vi "U8_3_byte_Array_with_dividor.vi"(10 "Array In":u8[](array[numeric]), 11 "Nmbr_of_datasamples":dbl=128.0) -> (0 "Current":dbl[](graph), 1 "mV":dbl, 2 "Voltage":dbl[](graph), 3 "Loop count":dbl, 4 "COM":dbl[](graph), 6 "HEXVAL":string)   [LabVIEW 2012]
panel:
  out "Dividor Value":dbl[](array[numeric])
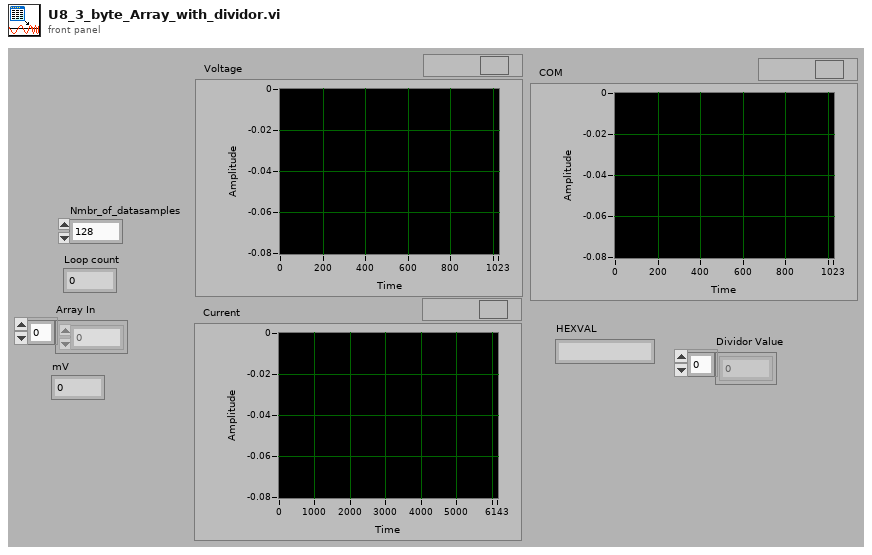
[diagram p1: front panel]
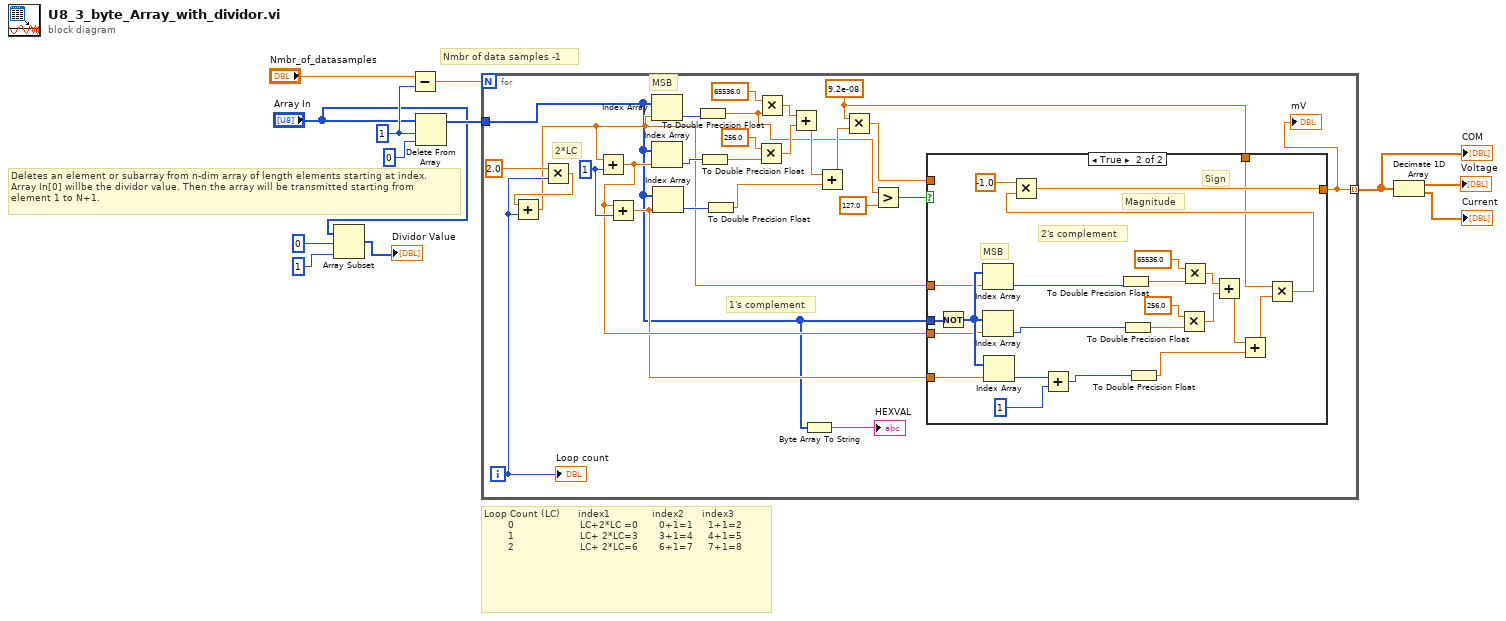
[diagram p0: block diagram]
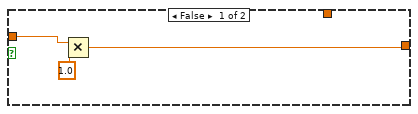
[diagram p2: hidden frame]
diagram:
  w5 = 1
  # "Nmbr of data samples -1"
  # "Deletes an element or subarray from n-dim array of length elements starting at index.\nArray In[0] willbe the dividor value. Then the array will be transmitted starting from\nelement 1 to N+1."
  # "Loop Count (LC)      index1              index2      index3      \n        0                      LC+2*LC =0       0+1=1     1+1=2\n        1                      LC+ 2*LC=3       3+1=4     4+1=5\n        2                      LC+ 2*LC=6       6+1=7     7+1=8"
  n1 = Array Subset(array="Array In", index=0, length=1) -> (→"Dividor Value":u8[])
  n2 = Subtract(x="Nmbr_of_datasamples", y=w5) -> (x-y=w11:dbl)
  n3 = Delete From Array(array="Array In", length=w5, index=0) -> (array with subset deleted=w9:u8[])  [unwired: 1 out]
  n4 = for {
    N: w11 -> [_]
    tunnel: w9 -> [w13]
    tunnel: [w15] -> w6 mode=indexing
    i -> [w20]
    w19 = 9.2e-08
    w30 = 1
    # "1's complement"
    # "MSB"
    # "2*LC"
    n5 = Multiply(x=2.0, y=w20) -> (x*y=w28:dbl)
    n6 = Add(x=w28, y=w20) -> (x+y=w18:dbl)
    n7 = Add(x=w18, y=w30) -> (x+y=w17:dbl)
    n8 = Add(x=w17, y=w30) -> (x+y=w16:dbl)
    n9 = Index Array(array=w13, index=w18) -> (element=w23:u8)
    n10 = Index Array(array=w13, index=w17) -> (element=w22:u8)
    n11 = Index Array(array=w13, index=w16) -> (element=w21:u8)
    n12 = To Double Precision Float(number=w23) -> (double precision float=w24:dbl)
    n13 = To Double Precision Float(number=w22) -> (double precision float=w36:dbl)
    n14 = To Double Precision Float(number=w21) -> (double precision float=w32:dbl)
    n15 = Multiply(x=256.0, y=w36) -> (x*y=w34:dbl)
    n16 = Multiply(x=65536.0, y=w24) -> (x*y=w38:dbl)
    n17 = Add(x=w38, y=w34) -> (x+y=w33:dbl)
    n18 = Byte Array To String(unsigned byte array=w13) -> (string=→"HEXVAL":string)
    n19 = Add(x=w33, y=w32) -> (x+y=w31:dbl)
    n20 = Multiply(x=w19, y=w31) -> (x*y=w27:dbl)
    n21 = Greater?(x=w24, y=127.0) -> (0:w26:bool)
    n22 = case shown="True" w26 {
      tunnel: [w41 w64] -> w15
      tunnel: w27 -> [w40 _]
      tunnel: w13 -> [_ w51]
      tunnel: w18 -> [_ w46]
      tunnel: w17 -> [_ w45]
      tunnel: w16 -> [_ w44]
      tunnel: w19 -> [_ w42]
      frame False {
        n23 = Multiply(x=w40, y=1.0) -> (x*y=w41:dbl)
      }
      frame True {
        # "Magnitude"
        # "Sign"
        # "2's complement"
        # "MSB"
        n24 = Not(x=w51) -> (.not. x?=w50:u8[])
        n25 = Index Array(array=w50, index=w46) -> (element=w53:u8)
        n26 = Index Array(array=w50, index=w45) -> (element=w52:u8)
        n27 = Index Array(array=w50, index=w44) -> (element=w49:u8)
        n28 = Add(x=w49, y=1) -> (x+y=w47:i32)
        n29 = To Double Precision Float(number=w53) -> (double precision float=w54:dbl)
        n30 = To Double Precision Float(number=w52) -> (double precision float=w60:dbl)
        n31 = To Double Precision Float(number=w47) -> (double precision float=w56:dbl)
        n32 = Multiply(x=256.0, y=w60) -> (x*y=w58:dbl)
        n33 = Multiply(x=65536.0, y=w54) -> (x*y=w62:dbl)
        n34 = Add(x=w62, y=w58) -> (x+y=w57:dbl)
        n35 = Add(x=w57, y=w56) -> (x+y=w55:dbl)
        n36 = Multiply(x=w42, y=w55) -> (x*y=w43:dbl)
        n37 = Multiply(x=-1.0, y=w43) -> (x*y=w64:dbl)
      }
    }
    "mV" <- w15
    "Loop count" <- w20
  }
  "COM" <- w6
  n38 = Decimate 1D Array(w6) -> (→"Voltage":dbl[], →"Current":dbl[])
